vi "DeleteUser.vi"(8 "index":i32, 11 "UserLibFile":path) -> ()   [LabVIEW 2020]
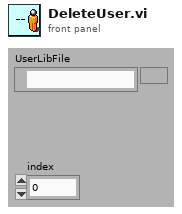
[diagram p1: front panel]
types:
  T1 = enum16{"open", "replace", "create", "open or create", "replace or create", "replace or create with confirmation"}
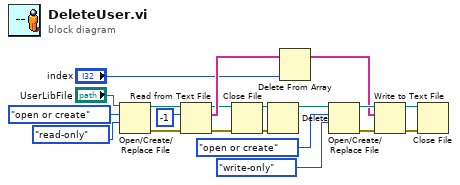
[diagram p0: block diagram]
diagram:
  n1 = Open/Create/Replace File(file path (use dialog)="UserLibFile", operation (0:open)=T1."open or create", access (0:read/write)=enum16{"read/write", "read-only", "write-only"}."read-only") -> (refnum out=w18:refnum<file>, error out=w17:errorcluster)  [unwired: 1 in, 3 out]
  n2 = Read from Text File(file (use dialog)=w18, count=-1, error in=w17) -> (refnum out=w14:refnum<file>, text=w15:string[], error out=w13:errorcluster)  [unwired: 2 out]
  n3 = Close File(refnum=w14, error in=w13) -> (path=w5:path, error out=w6:errorcluster)
  n4 = Delete(path (use dialog)=w5, error in=w6) -> (deleted path=w4:path)  [unwired: 5 out]
  n5 = Delete From Array(array=w15, index="index") -> (array with subset deleted=w2:string[])  [unwired: 1 in, 1 out]
  n6 = Open/Create/Replace File(file path (use dialog)=w4, operation (0:open)=T1."open or create", access (0:read/write)=enum16{"read/write", "read-only", "write-only"}."write-only") -> (refnum out=w9:refnum<file>, error out=w10:errorcluster)  [unwired: 1 in, 3 out]
  n7 = Write to Text File(file (use dialog)=w9, text=w2, error in=w10) -> (refnum out=w7:refnum<file>, error out=w8:errorcluster)  [unwired: 2 out]
  n8 = Close File(refnum=w7, error in=w8) -> ()  [unwired: 2 out]
